vi "Event Handle Loop_Set Page Attribute.vi"(8 "error in (no error)":errorcluster, 10 "Pag Attribute":T1, 11 "QTab Class in":refnum<class "QTab Class.lvclass">) -> (0 "error out":errorcluster, 3 "QTab Class out":refnum<class "QTab Class.lvclass">)   [LabVIEW 2020, in "QTab.lvlib" / "QTab Class.lvclass"]
uses:
  QTab Class.lvclass
  Pag Attribute.ctl
  QTab Class.lvclass/QTab Class.ctl
  QMenu Class/Button Attribute.ctl
  QMenu Class/QMenu Class.lvclass
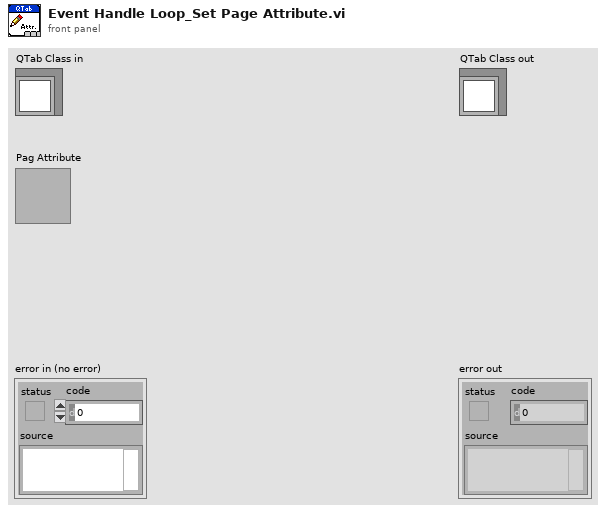
[diagram p1: front panel]
types:
  T1 = typedef "QTab.lvlib/QTab Class.lvclass/Pag Attribute.ctl" = cluster{"VI Refnum":refnum<vi>, "Page Name":string, "Closeable":bool, "Draggable":bool, "Pop-Out":bool}
  T2 = typedef "QTab.lvlib/QMenu Class.lvclass/Button Attribute.ctl" = cluster{"Label":string, "Button Text":string, "Closable":bool, "Draggable":bool}
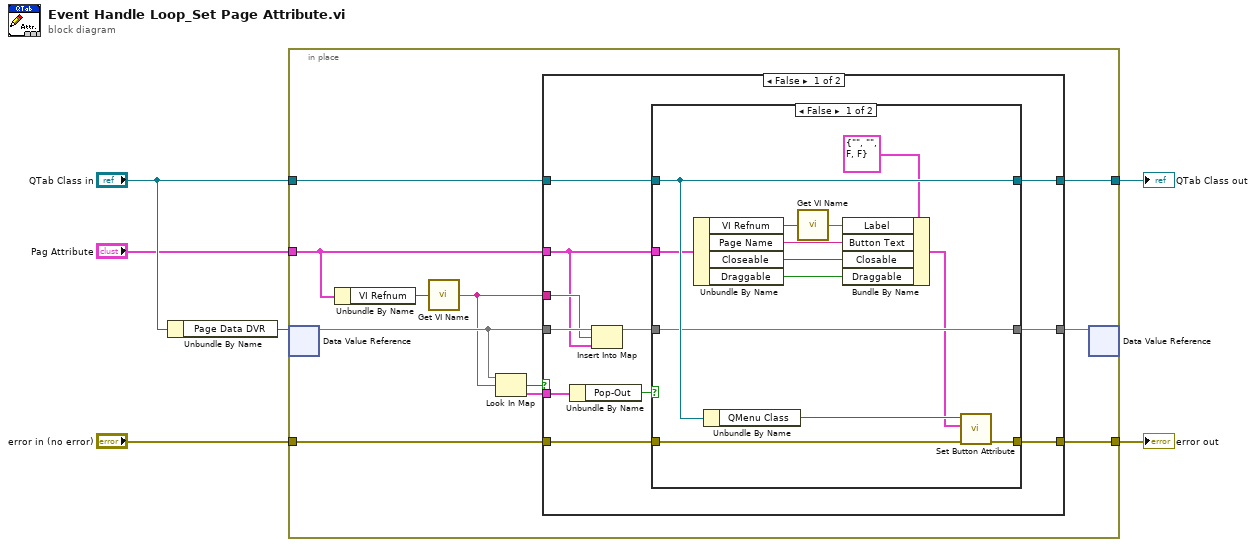
[diagram p0: block diagram]
diagram:
  n1 = Unbundle By Name("QTab Class in") -> ("Page Data DVR"=w6:refnum<data-value>)
  n2 = in-place {
    in-place-border: "Pag Attribute" -> [w16]
    in-place-border: "QTab Class in" -> [w15]
    in-place-border: "error in (no error)" -> [w9]
    in-place-border: [w14] -> w2
    in-place-border: [w10] -> w1
    n3 = in-place-dvr #1(w6) -> (w13:map{string, T1})  [unwired: 1 out]
    n4 = Unbundle By Name(w16) -> ("VI Refnum"=w8:refnum<vi>)
    n5 = call "Get VI Name.vi"("VI Refnum"=w8) -> ("VI Name"=w7:string)
    n6 = Look In Map(map=w13, key=w7) -> (key not found?=w17:bool, value=w11:T1)  [unwired: 1 in]
    n7 = case shown="False" w17 {
      tunnel: w9 -> [w19 w45]
      tunnel: w16 -> [w20 _]
      tunnel: w15 -> [w24 w47]
      tunnel: [w23 w47] -> w14
      tunnel: w13 -> [w28 w46]
      tunnel: [w21 w46] -> w12
      tunnel: w7 -> [w27 _]
      tunnel: w11 -> [w26 _]
      tunnel: [w18 w45] -> w10
      frame False {
        n8 = Unbundle By Name(w26) -> ("Pop-Out"=w25:bool)
        n9 = Insert Into Map(map in=w28, key=w27, value=w20) -> (map out=w22:map{string, T1})  [unwired: 2 out]
        n10 = case shown="False" w25 {
          tunnel: w24 -> [w41 w44]
          tunnel: [w41 w44] -> w23
          tunnel: w22 -> [w37 w43]
          tunnel: [w37 w43] -> w21
          tunnel: w20 -> [w35 _]
          tunnel: w19 -> [w39 w42]
          tunnel: [w38 w42] -> w18
          frame False {
            n11 = Unbundle By Name(w35) -> ("VI Refnum"=w30:refnum<vi>, "Page Name"=w34:string, "Closeable"=w33:bool, "Draggable"=w32:bool)
            n12 = Unbundle By Name(w41) -> ("QMenu Class"=w40:refnum<class "QMenu Class.lvclass">)
            n13 = call "Get VI Name.vi"("VI Refnum"=w30) -> ("VI Name"=w29:string)
            n14 = Bundle By Name(cluster=T2 {"Label"="", "Button Text"="", "Closable"=FALSE, "Draggable"=FALSE} ("Button Attribute"), "Label"=w29, "Button Text"=w34, "Closable"=w33, "Draggable"=w32) -> (w31:T2)
            n15 = call "Set Button Attribute.vi"("error in (no error)"=w39, "Button Attribute"=w31, "QMenu Class in"=w40) -> ("error out"=w38:errorcluster)  [unwired: 7 in, 1 out]
          }
          frame True {
          }
        }
      }
      frame True {
      }
    }
    n16 = in-place-dvr #1(w12) -> ()  [unwired: 2 out]
  }
  "error out" <- w1
  "QTab Class out" <- w2
